vi "Day 16-Recurse Packets.vi"(11 "String":string) -> (1 "Sum of Versions":u64, 2 "Return Value":u64, 3 "Left over bits":string)   [LabVIEW 2021]
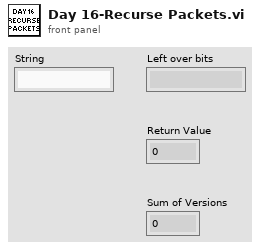
[diagram p1: front panel]
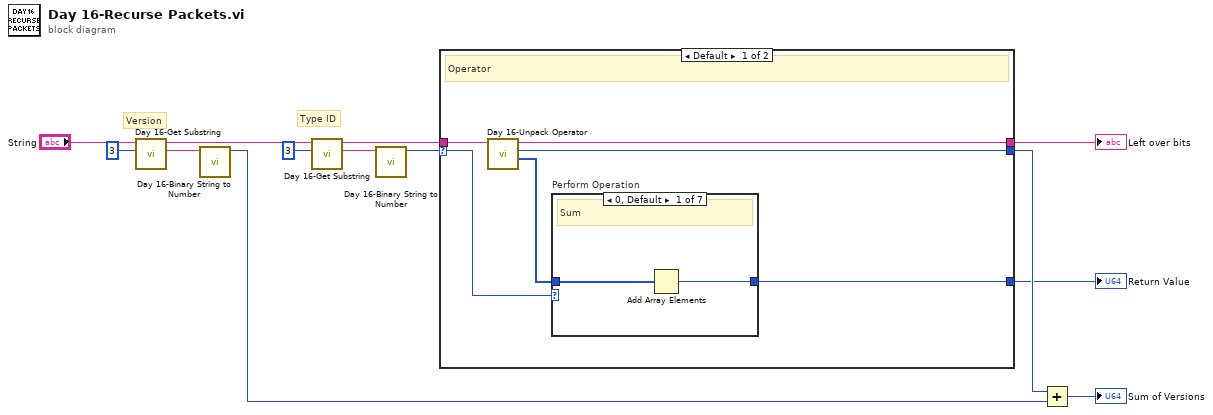
[diagram p0: block diagram]
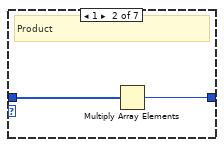
[diagram p2: hidden frame]
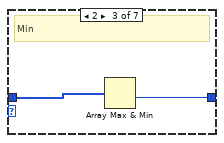
[diagram p3: hidden frame]
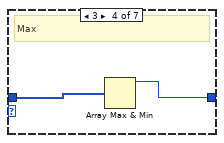
[diagram p4: hidden frame]
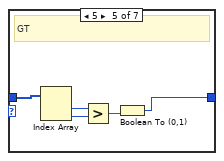
[diagram p5: hidden frame]
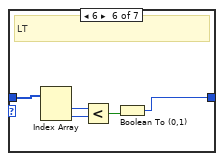
[diagram p6: hidden frame]
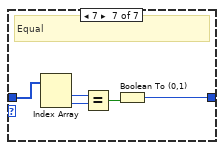
[diagram p7: hidden frame]
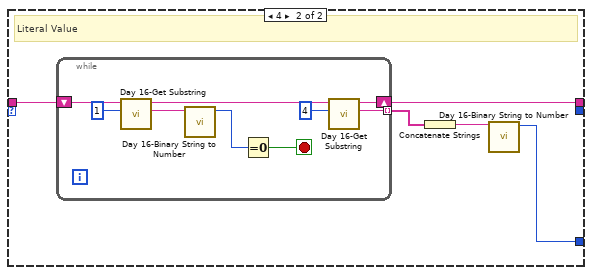
[diagram p8: hidden frame]
diagram:
  # "Type ID"
  # "Version"
  n1 = call "Day 16-Get Substring.vi"("length"=3, "String in"="String") -> ("Substring"=w4:string, "String out"=w9:string)  [unwired: 8 in]
  n2 = call "Day 16-Binary String to Number.vi"("Substring"=w4) -> ("Numeric"=w3:u64)  [unwired: 10 in]
  n3 = call "Day 16-Get Substring.vi"("length"=3, "String in"=w9) -> ("Substring"=w2:string, "String out"=w8:string)  [unwired: 8 in]
  n4 = call "Day 16-Binary String to Number.vi"("Substring"=w2) -> ("Numeric"=w1:u64)  [unwired: 10 in]
  n5 = case shown="Default" w1 {
    selector: w1 -> [w17 _]
    tunnel: w8 -> [w19 w47]
    tunnel: [w18 w46] -> w6
    tunnel: [w14 _] -> w7
    tunnel: [w16 w43] -> w5
    frame Default {
      # "Operator"
      n6 = call "Day 16-Unpack Operator.vi"("String in"=w19) -> ("Results Array"=w15:u64[], "Sum of Versions"=w14:u64, "String out"=w18:string)  [unwired: 8 in]
      n7 = case "Perform Operation" shown="0, Default" w17 {
        tunnel: w15 -> [w21 w23 w25 w27 w32 w37 w42]
        tunnel: [w20 w22 w24 w26 w28 w33 w38] -> w16
        frame 0, Default {
          # "Sum"
          n8 = Add Array Elements(numeric array=w21) -> (sum=w20:u64)
        }
        frame 1 {
          # "Product"
          n9 = Multiply Array Elements(1:w23) -> (0:w22:u64)
        }
        frame 2 {
          # "Min"
          n10 = Array Max & Min(array=w25) -> (min value=w24:u64)  [unwired: 3 out]
        }
        frame 3 {
          # "Max"
          n11 = Array Max & Min(array=w27) -> (max value=w26:u64)  [unwired: 3 out]
        }
        frame 5 {
          # "GT"
          n12 = Index Array(array=w32) -> (element #1=w31:u64, element #2=w30:u64)  [unwired: 2 in]
          n13 = Greater?(x=w31, y=w30) -> (0:w29:bool)
          n14 = Boolean To (0,1)(Boolean=w29) -> (0, 1=w28:i16)
        }
        frame 6 {
          # "LT"
          n15 = Index Array(array=w37) -> (element #1=w36:u64, element #2=w35:u64)  [unwired: 2 in]
          n16 = Less?(x=w36, y=w35) -> (x < y?=w34:bool)
          n17 = Boolean To (0,1)(Boolean=w34) -> (0, 1=w33:i16)
        }
        frame 7 {
          # "Equal"
          n18 = Index Array(array=w42) -> (element #1=w41:u64, element #2=w40:u64)  [unwired: 2 in]
          n19 = Equal?(x=w41, y=w40) -> (x = y?=w39:bool)
          n20 = Boolean To (0,1)(Boolean=w39) -> (0, 1=w38:i16)
        }
      }
    }
    frame 4 {
      # "Literal Value"
      n21 = while {
        shift-right: [w52] -> w46
        shift-left: w47 -> [w55]
        tunnel: [w50] -> w45 mode=indexing
        stop <- w51 stop-if-true
        n22 = call "Day 16-Get Substring.vi"("length"=1, "String in"=w55) -> ("Substring"=w49:string, "String out"=w53:string)  [unwired: 8 in]
        n23 = call "Day 16-Binary String to Number.vi"("Substring"=w49) -> ("Numeric"=w48:u64)  [unwired: 10 in]
        n24 = Equal To 0?(x=w48) -> (x = 0?=w51:bool)
        n25 = call "Day 16-Get Substring.vi"("length"=4, "String in"=w53) -> ("Substring"=w50:string, "String out"=w52:string)  [unwired: 8 in]
      }
      n26 = Concatenate Strings(w45) -> (w44:string)
      n27 = call "Day 16-Binary String to Number.vi"("Substring"=w44) -> ("Numeric"=w43:u64)  [unwired: 10 in]
    }
  }
  "Left over bits" <- w6
  "Return Value" <- w5
  n28 = Add(x=w7, y=w3) -> (x+y=→"Sum of Versions":u64)
